vi "pharosControl.vi"() -> ()   [LabVIEW 2017]
uses:
  <vilib>/DAQmx/write.llb/DAQmx Write (Digital 1D U8 1Chan NSamp).vi
  <vilib>/DAQmx/write.llb/DAQmx Write (Digital U8 1Chan 1Samp).vi
  globalDevices.vi
  globalUtilities.vi
  <vilib>/DAQmx/miscellaneous.llb/DAQmx Fill In Error Info.vi
panel:
  in  "pharosTimeBtwTrains":dbl
  in  "pharosNTrains":i32=1
  in  "const. duration":bool
  in  "allowExtCtrl":bool
  out "time elapsed":dbl format="%.2f"
  in  "total duration (s)":dbl
  out "interval between pulses (s)":dbl format="%.6f"
  in  "fire":bool
  in  "stop":bool
  in  "pharosNPulses":i32=500000 min=0
  in  "pharosRepRateDivider":i32=500 min=1 max=10000
  in  "mode":u16(ring) items=["static", "pulse train"]
  in  "on":bool
  # "(s)"
  # "THE CONTROL SOURCE OF THE\nPULSE PICKER SHOULD BE SET TO\nEXTERNAL IN THE PHAROS APP\n(FROM STAND-BY MODE)."
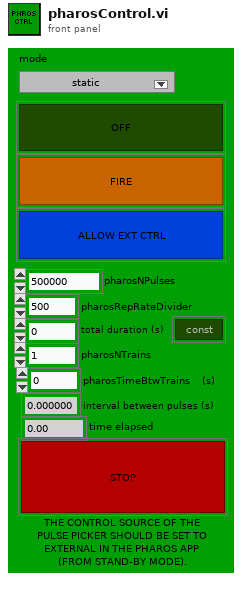
[diagram p1: front panel]
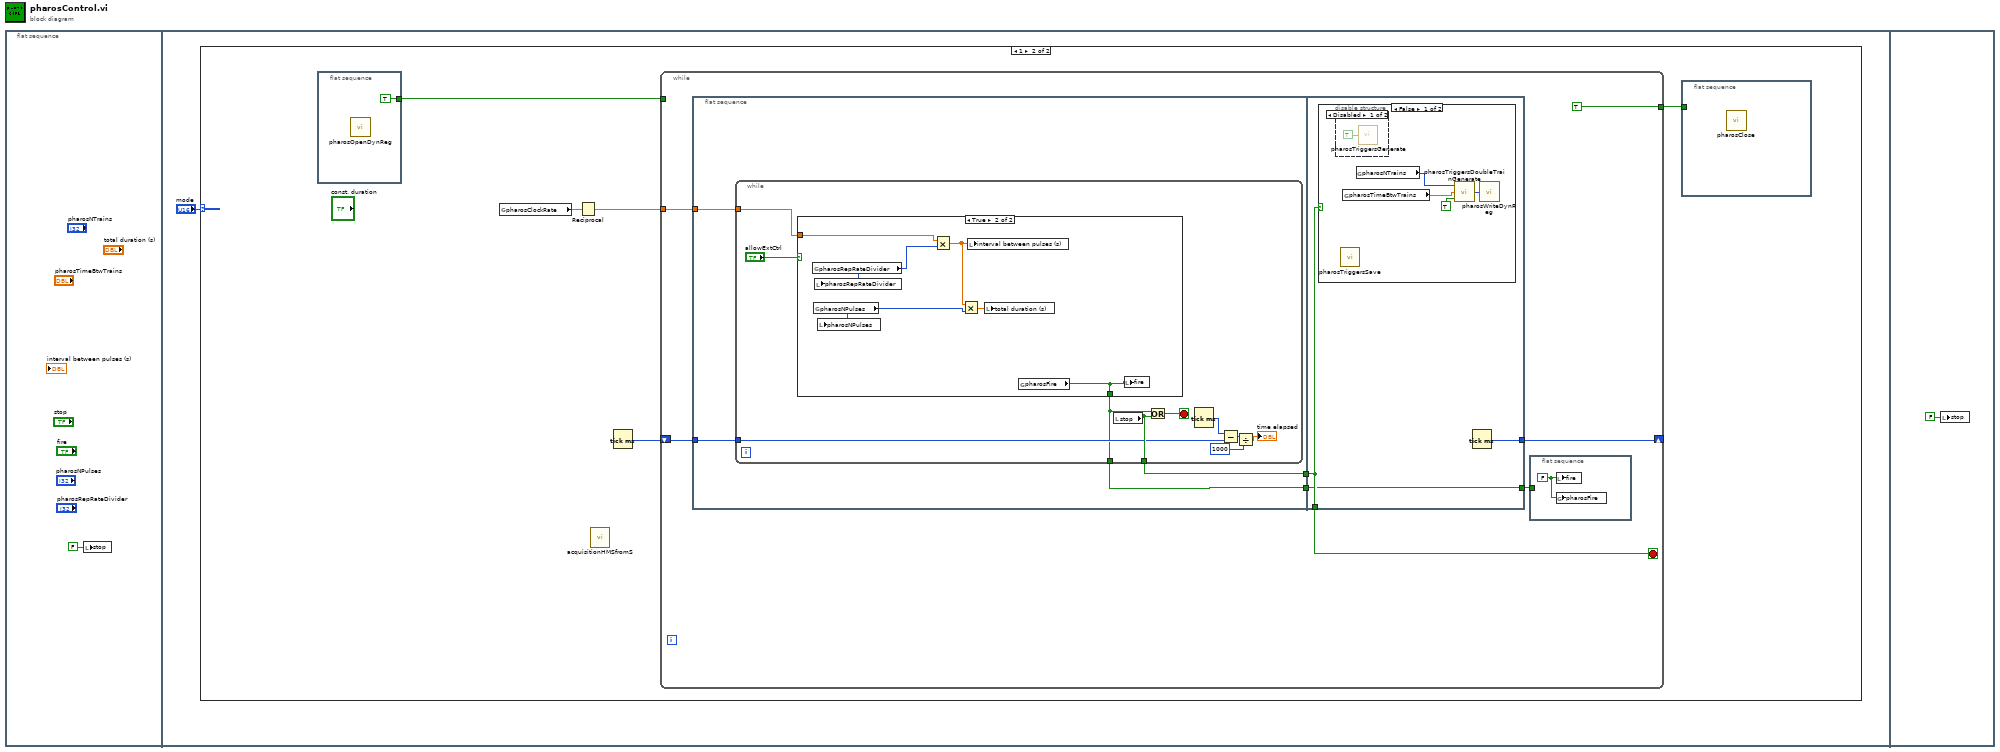
[diagram p0: block diagram]
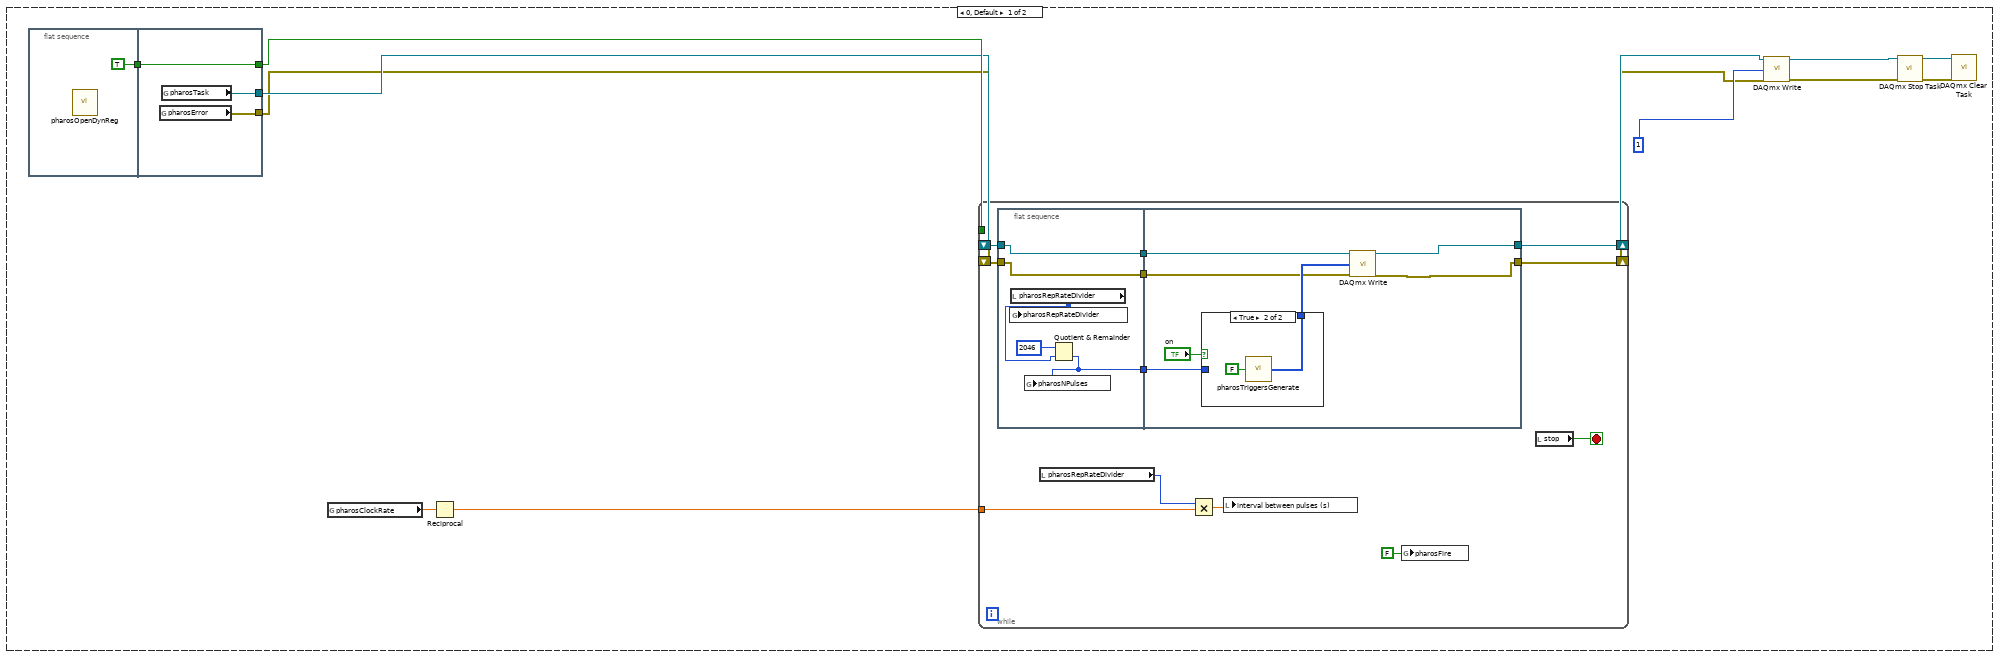
[diagram p2: hidden frame]
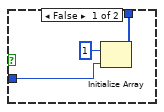
[diagram p3: hidden frame]
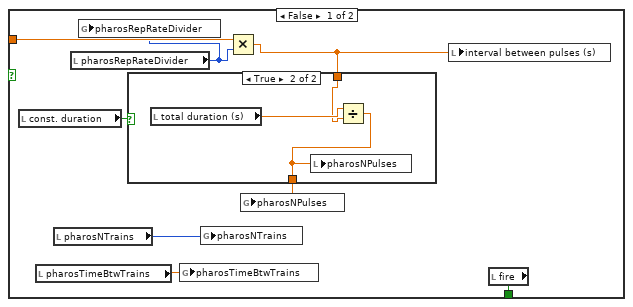
[diagram p4: hidden frame]
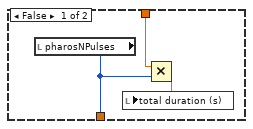
[diagram p5: hidden frame]
diagram:
  n1 = flat-sequence {
    frame #0 {
      n2 = local write "stop"(FALSE ("stop")) -> ()
    }
    frame #1 {
      n3 = case shown="1" "mode" {
        frame 0, Default {
          n4 = flat-sequence {
            tunnel: [TRUE] -> w9
            tunnel: [w19] -> w10
            tunnel: w9 -> [w19]
            tunnel: [w18] -> w8
            tunnel: [w17] -> w7
            frame #0 {
              n5 = call "pharosOpenDynReg.vi"() -> ()  [unwired: 12 in]
            }
            frame #1 {
              n6 = global read "globalDevices.vi" "pharosError"() -> (w17:errorcluster)
              n7 = global read "globalDevices.vi" "pharosTask"() -> (w18:refnum<k21>)
            }
          }
          n8 = global read "globalDevices.vi" "pharosClockRate"() -> (w4:dbl)
          n9 = Reciprocal(x=w4) -> (1/x=w3:dbl)
          n10 = while {
            tunnel: w10 -> [_]
            shift-right: [w26] -> w6
            shift-left: w8 -> [w30]
            shift-right: [w25] -> w5
            shift-left: w7 -> [w28]
            tunnel: w3 -> [w22]
            stop <- w31 stop-if-true
            n11 = flat-sequence {
              tunnel: w30 -> [w36]
              tunnel: [w36] -> w29
              tunnel: w28 -> [w35]
              tunnel: [w35] -> w27
              tunnel: [w32] -> w24
              tunnel: w29 -> [w41]
              tunnel: w27 -> [w40]
              tunnel: [w39] -> w26
              tunnel: [w38] -> w25
              tunnel: w24 -> [w37]
              frame #0 {
                n12 = local read "pharosRepRateDivider"() -> (w33:i32)
                n13 = global write "globalUtilities.vi" "pharosRepRateDivider"(w33) -> ()
                n14 = Quotient & Remainder(x=2046 ("pharosNPulses"), y=w33) -> (floor(x/y)=w32:i32)  [unwired: 1 out]
                n15 = global write "globalUtilities.vi" "pharosNPulses"(w32) -> ()
              }
              frame #1 {
                n16 = case shown="True" "on" {
                  tunnel: [w45 w47] -> w42
                  tunnel: w37 -> [w44 _]
                  frame False {
                    n17 = Initialize Array(u8 1 ("element"), w44) -> (w45:u8[])
                  }
                  frame True {
                    n18 = call "pharosTriggersGenerate.vi"("off at the end"=FALSE) -> ("triggers"=w47:u8[])
                  }
                }
                n19 = call-poly <vilib>:"DAQmx Write.vi"("task/channels in"=w41, "data"=w42, "error in"=w40) -> ("task out"=w39:refnum<k21>, "error out"=w38:errorcluster)  [unwired: 10 in, 1 out]
              }
            }
            n20 = local read "pharosRepRateDivider"() -> (w23:i32)
            n21 = Multiply(x=w23, y=w22) -> (x*y=w21:dbl)
            n22 = local write "interval between pulses (s)"(w21) -> ()
            n23 = global write "globalUtilities.vi" "pharosFire"(FALSE ("pharosFire")) -> ()
            n24 = local read "stop"() -> (w31:bool)
          }
          n25 = call-poly <vilib>:"DAQmx Write.vi"("task/channels in"=w6, "data"=u8 1, "error in"=w5) -> ("task out"=w12:refnum<k21>, "error out"=w11:errorcluster)  [unwired: 10 in, 1 out]
          n26 = call <vilib>:"DAQmx Stop Task.vi"("task/channels in"=w12, "error in"=w11) -> ("task out"=w13:refnum<k21>, "error out"=w14:errorcluster)  [unwired: 12 in]
          n27 = call <vilib>:"DAQmx Clear Task.vi"("task in"=w13, "error in"=w14) -> ()  [unwired: 13 in, 1 out]
        }
        frame 1 {
          n28 = flat-sequence {
            tunnel: [TRUE] -> w53
            frame #0 {
              n29 = call "pharosOpenDynReg.vi"() -> ()  [unwired: 12 in]
            }
          }
          n30 = global read "globalDevices.vi" "pharosClockRate"() -> (w49:dbl)
          n31 = Reciprocal(x=w49) -> (1/x=w51:dbl)
          n32 = call "acquisitionHMSfromS.vi"() -> ()  [unwired: 1 in, 4 out]
          n33 = Tick Count (ms)() -> (millisecond timer value=w50:u32)
          n34 = while {
            tunnel: w53 -> [_]
            tunnel: [TRUE] -> w52
            tunnel: w51 -> [w57]
            shift-right: [w55] -> _
            shift-left: w50 -> [w56]
            stop <- w61 stop-if-true
            n35 = flat-sequence {
              tunnel: [w67] -> w62
              tunnel: [w66] -> w60
              tunnel: w57 -> [w65]
              tunnel: w56 -> [w64]
              tunnel: w62 -> [w100]
              tunnel: [w100] -> w61
              tunnel: w60 -> [w99]
              tunnel: [w99] -> w59
              tunnel: [w98] -> w55
              frame #0 {
                n36 = while {
                  tunnel: [w76] -> w67
                  tunnel: [w69] -> w66
                  tunnel: w65 -> [w68]
                  tunnel: w64 -> [w74]
                  stop <- w77 stop-if-true
                  n37 = case shown="True" "allowExtCtrl" {
                    tunnel: [w85 w97] -> w69
                    tunnel: w68 -> [w82 w96]
                    frame False {
                      n38 = local read "const. duration"() -> (w84:bool)
                      n39 = local read "pharosTimeBtwTrains"() -> (w78:dbl)
                      n40 = local read "pharosNTrains"() -> (w79:i32)
                      n41 = local read "pharosRepRateDivider"() -> (w80:i32)
                      n42 = global write "globalUtilities.vi" "pharosRepRateDivider"(w80) -> ()
                      n43 = global write "globalUtilities.vi" "pharosTimeBtwTrains"(w78) -> ()
                      n44 = global write "globalUtilities.vi" "pharosNTrains"(w79) -> ()
                      n45 = Multiply(x=w82, y=w80) -> (x*y=w81:dbl)
                      n46 = case shown="True" w84 {
                        tunnel: [w87 w91] -> w83
                        tunnel: w81 -> [w86 w89]
                        frame False {
                          n47 = local read "pharosNPulses"() -> (w87:i32)
                          n48 = Multiply(x=w86, y=w87) -> (x*y=w88:dbl)
                          n49 = local write "total duration (s)"(w88) -> ()
                        }
                        frame True {
                          n50 = local read "total duration (s)"() -> (w90:dbl)
                          n51 = Divide(x=w90, y=w89) -> (x/y=w91:dbl)
                          n52 = local write "pharosNPulses"(w91) -> ()
                        }
                      }
                      n53 = global write "globalUtilities.vi" "pharosNPulses"(w83) -> ()
                      n54 = local write "interval between pulses (s)"(w81) -> ()
                      n55 = local read "fire"() -> (w85:bool)
                    }
                    frame True {
                      n56 = global read "globalUtilities.vi" "pharosRepRateDivider"() -> (w95:i32)
                      n57 = global read "globalUtilities.vi" "pharosNPulses"() -> (w93:i32)
                      n58 = local write "pharosRepRateDivider"(w95) -> ()
                      n59 = local write "pharosNPulses"(w93) -> ()
                      n60 = Multiply(x=w96, y=w95) -> (x*y=w94:dbl)
                      n61 = Multiply(x=w94, y=w93) -> (x*y=w92:dbl)
                      n62 = local write "interval between pulses (s)"(w94) -> ()
                      n63 = local write "total duration (s)"(w92) -> ()
                      n64 = global read "globalUtilities.vi" "pharosFire"() -> (w97:bool)
                      n65 = local write "fire"(w97) -> ()
                    }
                  }
                  n66 = local read "stop"() -> (w76:bool)
                  n67 = Or(x=w69, y=w76) -> (x .or. y?=w77:bool)
                  n68 = Tick Count (ms)() -> (millisecond timer value=w75:u32)
                  n69 = Subtract(x=w75, y=w74) -> (x-y=w73:u32)
                  n70 = Divide(x=w73, y=u32 1000) -> (x/y=→"time elapsed":dbl)
                }
              }
              frame #1 {
                n71 = case shown="False" w100 {
                  frame False {
                    n72 = disable-structure shown="Disabled" {
                      frame Disabled {
                        n73 = call "pharosTriggersGenerate.vi"("off at the end"=TRUE) -> ()  [unwired: 1 out]
                      }
                      frame Enabled {
                      }
                    }
                    n74 = call "pharosTriggersSave.vi"() -> ()  [unwired: 2 in]
                    n75 = global read "globalUtilities.vi" "pharosTimeBtwTrains"() -> (w101:dbl)
                    n76 = global read "globalUtilities.vi" "pharosNTrains"() -> (w102:i32)
                    n77 = call "pharosTriggersDoubleTrainGenerate.vi"("off at the end"=TRUE, "time btwn trains (s)"=w101, "n trains"=w102) -> ("triggers"=w104:u8[])
                    n78 = call "pharosWriteDynReg.vi"("triggers"=w104) -> ()  [unwired: 1 in]
                  }
                  frame True {
                  }
                }
                n79 = Tick Count (ms)() -> (millisecond timer value=w98:u32)
              }
            }
            n80 = flat-sequence {
              tunnel: w59 -> [_]
              frame #0 {
                w63 = FALSE ("fire")
                n81 = local write "fire"(w63) -> ()
                n82 = global write "globalUtilities.vi" "pharosFire"(w63) -> ()
              }
            }
          }
          n83 = flat-sequence {
            tunnel: w52 -> [_]
            frame #0 {
              n84 = call "pharosClose.vi"() -> ()  [unwired: 12 in]
            }
          }
        }
      }
    }
    frame #2 {
      n85 = local write "stop"(FALSE ("stop")) -> ()
    }
  }
